vi "CRYCheck Time Option.vi"(9 "Option Array In":bool[](array[boolean]), 10 "Averaging":u16, 11 "Algorithm":u16) -> (3 "Option Array Out":bool[](array[boolean]))   [LabVIEW 2013]
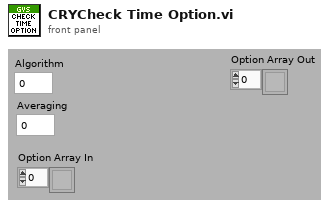
[diagram p1: front panel]
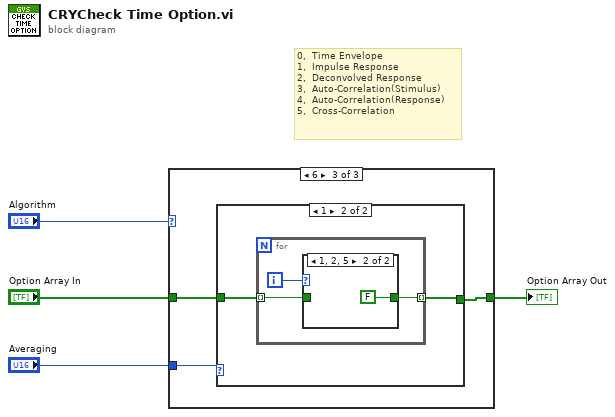
[diagram p0: block diagram]
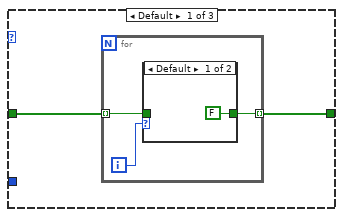
[diagram p2: hidden frame]
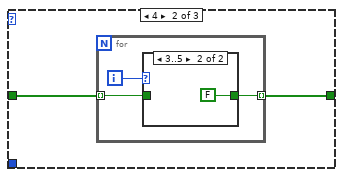
[diagram p4: hidden frame]
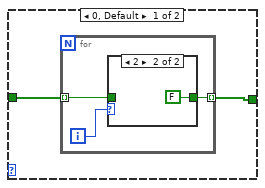
[diagram p6: hidden frame]
diagram:
  # "0,  Time Envelope\n1,  Impulse Response\n2,  Deconvolved Response\n3,  Auto-Correlation(Stimulus)\n4,  Auto-Correlation(Response)\n5,  Cross-Correlation"
  n1 = case shown="6" "Algorithm" {
    tunnel: "Option Array In" -> [w6 w13 w21]
    tunnel: "Averaging" -> [_ _ w20]
    tunnel: [w5 w12 w19] -> w1
    frame Default {
      n2 = for {
        tunnel: w6 -> [w8] mode=indexing
        tunnel: [w7] -> w5 mode=indexing
        i -> [w9]
        n3 = case shown="Default" w9 {
          tunnel: [FALSE ("Is Har meas.freq? 2") w11] -> w7
          tunnel: w8 -> [_ w11]
          frame Default {
          }
          frame 0 {
          }
        }
      }
    }
    frame 4 {
      n4 = for {
        tunnel: w13 -> [w15] mode=indexing
        tunnel: [w14] -> w12 mode=indexing
        i -> [w16]
        n5 = case shown="3..5" w16 {
          tunnel: w15 -> [w17 _]
          tunnel: [w17 FALSE ("Is Har meas.freq? 2")] -> w14
          frame Default {
          }
          frame 3..5 {
          }
        }
      }
    }
    frame 6 {
      n6 = case shown="1" w20 {
        tunnel: w21 -> [w23 w30]
        tunnel: [w22 w29] -> w19
        frame 0, Default {
          n7 = for {
            tunnel: w23 -> [w25] mode=indexing
            tunnel: [w24] -> w22 mode=indexing
            i -> [w26]
            n8 = case shown="2" w26 {
              tunnel: [w27 FALSE ("Is Har meas.freq? 2")] -> w24
              tunnel: w25 -> [w27 _]
              frame Default {
              }
              frame 2 {
              }
            }
          }
        }
        frame 1 {
          n9 = for {
            tunnel: w30 -> [w32] mode=indexing
            tunnel: [w31] -> w29 mode=indexing
            i -> [w33]
            n10 = case shown="1, 2, 5" w33 {
              tunnel: w32 -> [w34 _]
              tunnel: [w34 FALSE ("Is Har meas.freq? 2")] -> w31
              frame Default {
              }
              frame 1, 2, 5 {
              }
            }
          }
        }
      }
    }
  }
  "Option Array Out" <- w1
